vi "TestStage.vi"() -> ()   [LabVIEW 2013]
uses:
  <vilib>/Utility/file.llb/Write To Spreadsheet File (DBL).vi
  <vilib>/express/express arith-compare/Formula/XNode/ExpressFormulaBlockNode.xnode
panel:
  out "iteration":dbl
  in  "speed":dbl
  out "currentPosition":dbl
  in  "Motor COM Port":refnum<visa-resource-name>="COM4"
  in  "Encoder COM Port":refnum<visa-resource-name>="COM1"
  in  "nRuns":i32
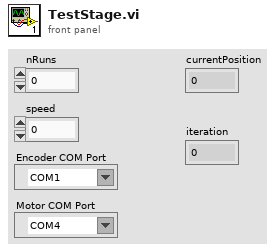
[diagram p1: front panel]
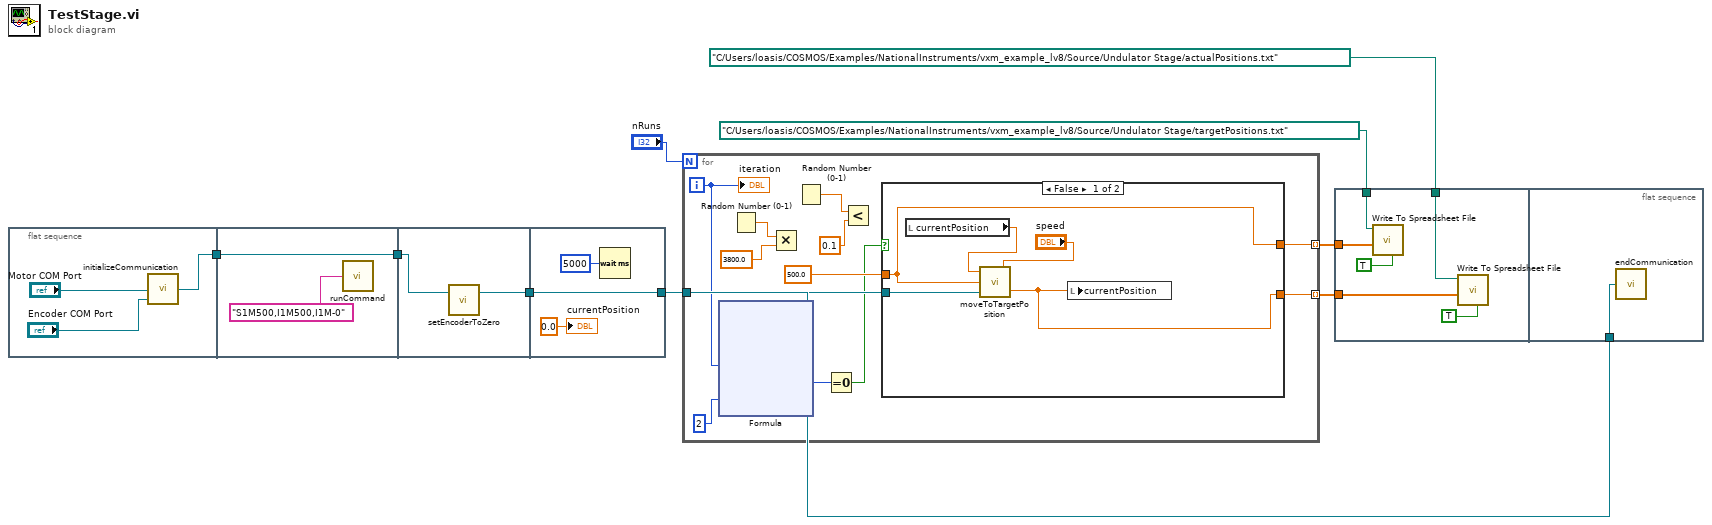
[diagram p0: block diagram]
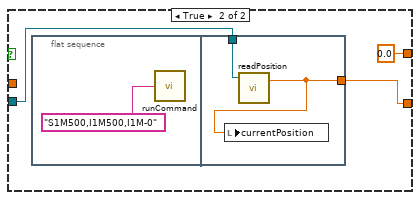
[diagram p2: hidden frame]
diagram:
  n1 = flat-sequence {
    tunnel: [w10] -> w7
    tunnel: [w13] -> w8
    tunnel: w7 -> [w13]
    tunnel: w8 -> [w16]
    tunnel: [w15] -> w6
    tunnel: [w19] -> w1
    tunnel: w6 -> [w19]
    frame #0 {
      n2 = call "initializeCommunication.vi"("Encoder COM Port"="Encoder COM Port", "Motor COM Port"="Motor COM Port") -> ("Encoder VISA Resource Name (out)"=w10:refnum<visa-resource-name>)  [unwired: 1 in]
    }
    frame #1 {
      n3 = call "runCommand.vi"("command"="S1M500,I1M500,I1M-0") -> ()  [unwired: 1 in]
    }
    frame #2 {
      n4 = call "setEncoderToZero.vi"("VISA resource name"=w16) -> ("VISA resource name out"=w15:refnum<visa-resource-name>)  [unwired: 1 in, 1 out]
    }
    frame #3 {
      n5 = Wait (ms)(milliseconds to wait=u32 5000) -> ()  [unwired: 1 out]
      "currentPosition" <- 0.0 ("currentPosition")
    }
  }
  n6 = for {
    N: "nRuns" -> [_]
    tunnel: w1 -> [w30]
    tunnel: [w27] -> w5 mode=indexing
    tunnel: [w26] -> w4 mode=indexing
    i -> [w20]
    n7 = xnode "Formula"("X1"=w20, "X2"=i8 2) -> ("Result"=w21:i32)  [unwired: 1 in, 1 out]
    n8 = Random Number (0-1)() -> (number: 0 to 1=w29:dbl)
    n9 = Multiply(x=w29, y=3800.0) -> ()  [unwired: 1 out]
    n10 = Random Number (0-1)() -> (number: 0 to 1=w25:dbl)
    n11 = Equal To 0?(x=w21) -> (x = 0?=w22:bool)
    n12 = Less?(x=w25, y=0.1) -> ()  [unwired: 1 out]
    n13 = case shown="False" w22 {
      tunnel: w30 -> [w46 w49]
      tunnel: 500.0 -> [w42 _]
      tunnel: [w43 w48] -> w26
      tunnel: [w42 0.0] -> w27
      frame False {
        n14 = local read "currentPosition"() -> (w45:dbl)
        n15 = call "moveToTargetPosition.vi"("speed"="speed", "Encoder COM Port"=w46, "targetPos"=w42, "currentPos"=w45) -> ("updatedCurrentPos"=w43:dbl)
        n16 = local write "currentPosition"(w43) -> ()
      }
      frame True {
        n17 = flat-sequence {
          tunnel: w49 -> [w52]
          tunnel: [w51] -> w48
          frame #0 {
            n18 = call "runCommand.vi"("command"="S1M500,I1M500,I1M-0") -> ()  [unwired: 1 in]
          }
          frame #1 {
            n19 = call "readPosition.vi"("VISA resource name"=w52) -> ("position"=w51:dbl)  [unwired: 1 in, 2 out]
            n20 = local write "currentPosition"(w51) -> ()
          }
        }
      }
    }
    "iteration" <- w20
  }
  n21 = flat-sequence {
    tunnel: w5 -> [w58]
    tunnel: w4 -> [w57]
    tunnel: path "C:/Users/loasis/COSMOS/Examples/NationalInstruments/vxm_example_lv8/Source/Undulator Stage/targetPositions.txt" ("file path (dialog if empty)") -> [w56]
    tunnel: path "C:/Users/loasis/COSMOS/Examples/NationalInstruments/vxm_example_lv8/Source/Undulator Stage/actualPositions.txt" ("file path (dialog if empty)") -> [w55]
    tunnel: w1 -> [w59]
    frame #0 {
      n22 = call-poly <vilib>:"Write To Spreadsheet File.vi"("transpose? (no:F)"=TRUE, "1D data"=w58, "file path (dialog if empty)"=w56) -> ()  [unwired: 5 in, 1 out]
      n23 = call-poly <vilib>:"Write To Spreadsheet File.vi"("transpose? (no:F)"=TRUE, "1D data"=w57, "file path (dialog if empty)"=w55) -> ()  [unwired: 5 in, 1 out]
    }
    frame #1 {
      n24 = call "endCommunication.vi"("Encoder COM Port"=w59) -> ()  [unwired: 1 in]
    }
  }
